vi "Filter Axis.vi"(0 "Graph Scale in":refnum<vi>[](array[refnum]), 7 "Coords":T1, 11 "error in":errorcluster, 12 "Bypass Filter":bool) -> (4 "Filter Graph Scale out":refnum<vi>[](array[refnum]), 8 "Axis Value":cluster{"X":dbl, "Y":dbl}[](array[cluster]), 15 "error out":errorcluster)   [LabVIEW 2023, in "ScrollZoomGraphChart.lvclass"]
uses:
  ScrollZoomGraphChart.lvclass
  <vilib>/Analysis/geometry.llb/Point in Polygon Position.ctl
  <vilib>/Analysis/NI_AAL_Geometry.lvlib
  <vilib>/Utility/miscctls.llb/LVPoint32TypeDef.ctl
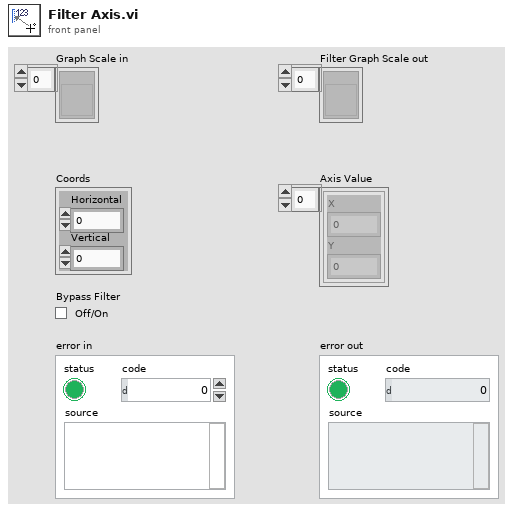
[diagram p1: front panel]
types:
  T1 = typedef "LVPoint32TypeDef.ctl" = cluster{"Horizontal":i32, "Vertical":i32}
  T2 = typedef "NI_AAL_Geometry.lvlib/Point in Polygon Position.ctl" = u16
  T3 = typedef "LVRectTypeDef.ctl" = cluster{"Left":i16, "Top":i16, "Right":i16, "Bottom":i16}
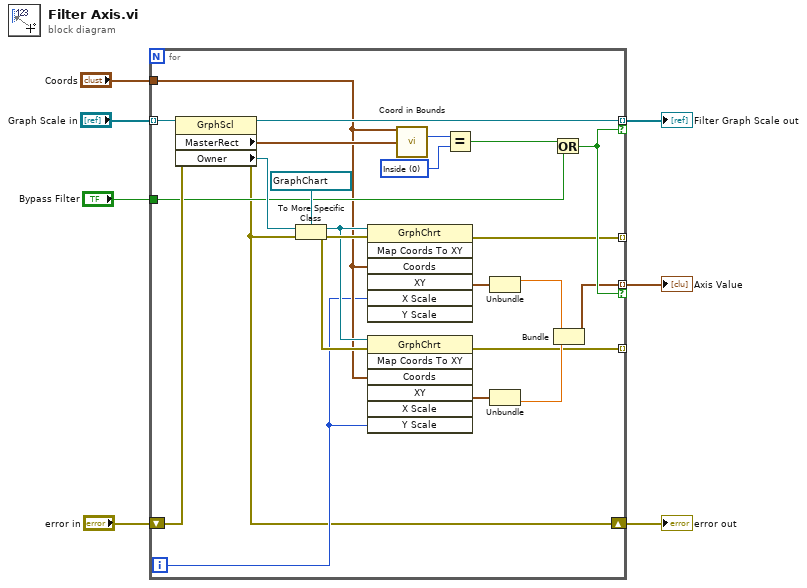
[diagram p0: block diagram]
diagram:
  n1 = for {
    tunnel: "Graph Scale in" -> [w29] mode=indexing
    tunnel: "Coords" -> [w17]
    tunnel: [w25] -> w5 mode=indexing if=w20
    tunnel: [w10] -> w2 mode=indexing if=w20
    shift-right: [w15] -> w3
    shift-left: "error in" -> [w22]
    tunnel: "Bypass Filter" -> [w19]
    tunnel: [w9] -> _ mode=indexing
    tunnel: [w8] -> _ mode=indexing
    i -> [w16]
    w26 = T2 0 items=["Inside", "On Boundary", "Outside"] ("x")
    n2 = property class="GrphScl"(reference=w29, error in=w22) -> (reference out=w25:refnum<vi>, error out=w15:errorcluster, "MasterRect"=w28:T3, "Owner"=w24:refnum<vi>)
    n3 = To More Specific Class(target class=refnum<vi> refnum ("reference"), reference=w24, error in=w15) -> (specific class reference=w18:refnum<vi>, error out=w30:errorcluster)
    n4 = invoke class="GrphChrt" method="Map Coords To XY"(reference=w18, error in=w30, "Coords"=w17, "X Scale"=w16) -> (error out=w9:errorcluster, "XY"=w14:cluster{"X":dbl, "Y":dbl})  [unwired: 3 in, 5 out]
    n5 = invoke class="GrphChrt" method="Map Coords To XY"(reference=w18, error in=w30, "Coords"=w17, "Y Scale"=w16) -> (error out=w8:errorcluster, "XY"=w13:cluster{"X":dbl, "Y":dbl})  [unwired: 3 in, 5 out]
    n6 = call "Coord in Bounds.vi"("Coords"=w17, "Plot Bounds"=w28) -> ("position"=w27:T2)  [unwired: 12 in, 1 out]
    n7 = Equal?(x=w27, y=w26) -> (x = y?=w21:bool)
    n8 = Unbundle(w14) -> ("X"=w12:dbl)  [unwired: 1 out]
    n9 = Unbundle(w13) -> ("Y"=w11:dbl)  [unwired: 1 out]
    n10 = Or(x=w21, y=w19) -> (x .or. y?=w20:bool)
    n11 = Bundle("X"=w12, "Y"=w11) -> (w10:cluster{"X":dbl, "Y":dbl})  [unwired: 1 in]
  }
  "Filter Graph Scale out" <- w5
  "error out" <- w3
  "Axis Value" <- w2
